vi "Unlock and limitDeg.vi"(2 "Timeout (ms)":i32=40000000, 3 "connection ID in":refnum<k5>) -> (0 "Timeout (ms) 2":i32=40000000, 1 "connection ID out":refnum<k5>)   [LabVIEW 2016]
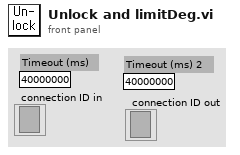
[diagram p1: front panel]
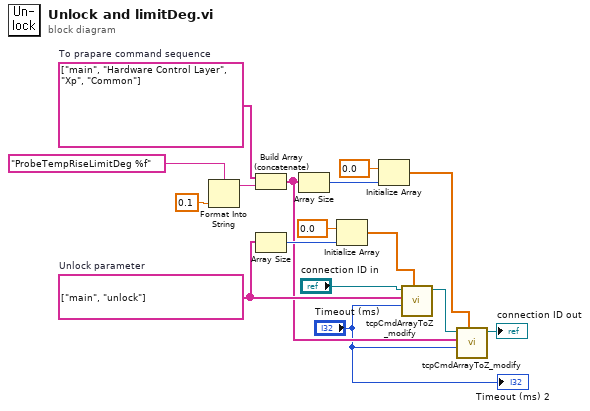
[diagram p0: block diagram]
diagram:
  w7 = string[] ["main", "Hardware Control Layer", "Xp", "Common"]  # To prapare command sequence
  w13 = string[] ["main", "unlock"]  # Unlock parameter
  n1 = Format Into String(format string="ProbeTempRiseLimitDeg %f", 0.1 ("입력 1")) -> (resulting string=w6:string)  [unwired: 2 in, 1 out]
  n2 = Build Array (concatenate)(w7, w6) -> (w5:string[])
  n3 = Array Size(array=w13) -> (size(s)=w16:i32)
  n4 = Array Size(array=w5) -> (size(s)=w12:i32)
  n5 = Initialize Array(0.0 ("element"), w16) -> (w14:dbl[])
  n6 = Initialize Array(0.0 ("element"), w12) -> (w10:dbl[])
  n7 = call "tcpCmdArrayToZ_modify.vi"("Delay (sec)"=w14, "Timeout (ms)"="Timeout (ms)", "Command array"=w13, "connection ID in"="connection ID in") -> ("connection ID out"=w4:refnum<k5>)  [unwired: 3 in, 4 out]
  n8 = call "tcpCmdArrayToZ_modify.vi"("Delay (sec)"=w10, "Timeout (ms)"="Timeout (ms)", "Command array"=w5, "connection ID in"=w4) -> ("connection ID out"=→"connection ID out":refnum<k5>)  [unwired: 3 in, 4 out]
  "Timeout (ms) 2" <- "Timeout (ms)"
